vi "Personality Test.vi"(0 "GEA2 Reference In":refnum<k24>, 5 "Model":string, 11 "error in (no error)":errorcluster) -> (3 "Personality":u8, 4 "GEA2 Reference Out":refnum<k24>, 6 "Report Text":string, 8 "Pass/Fail?":bool=TRUE, 10 "Model ID":u8, 14 "Version":string, 15 "Error Out":errorcluster)   [LabVIEW 2016]
doc: "This VI performs the personality test on the control. It reads the current personality stored and compares it to the expected personality for that particular model number. If they differ then it writes to change the model number to match the expected."
uses:
  C:/Automation/DLLs/PC Dot Net/GeaCommunication.dll
  Automation/DLLs/PC Dot Net/GeaCommunication.dll
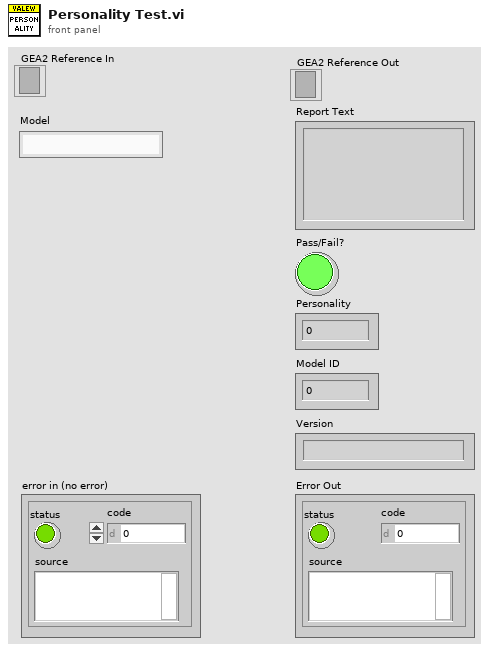
[diagram p1: front panel]
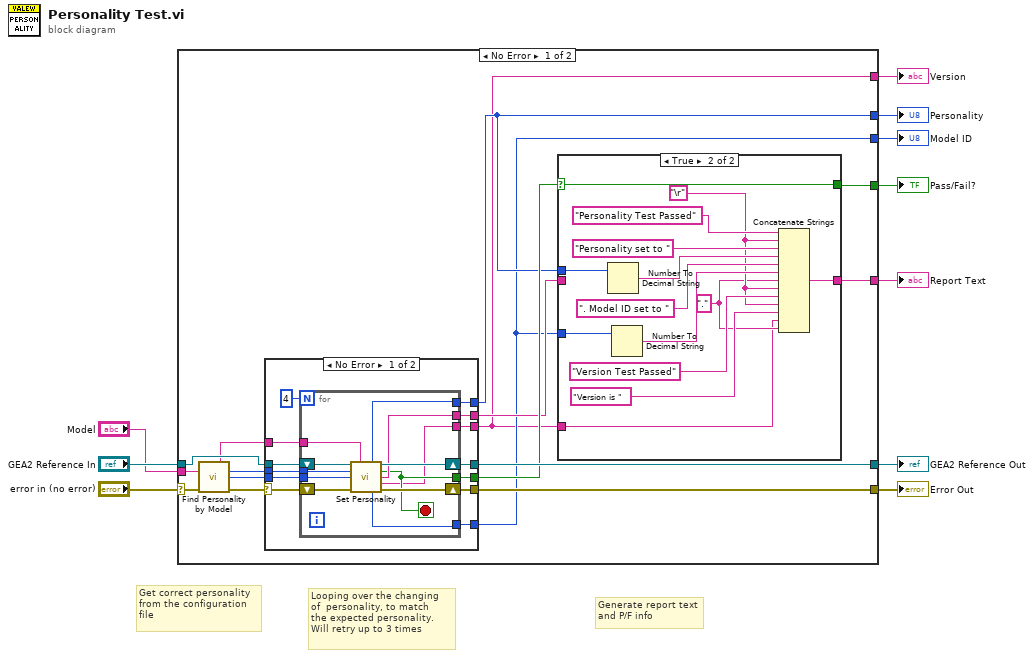
[diagram p0: block diagram]
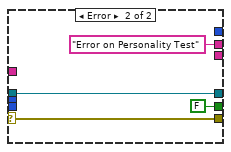
[diagram p2: hidden frame]
diagram:
  # "Generate report text\nand P/F info"
  # "Looping over the changing\nof  personality, to match \nthe expected personality. \nWill retry up to 3 times"
  # "Get correct personality\nfrom the configuration\nfile"
  n1 = case shown="No Error" "error in (no error)" {
    selector: "error in (no error)" -> [w18 w73]
    tunnel: [w26 w73] -> w10
    tunnel: "GEA2 Reference In" -> [w25 w72]
    tunnel: [w24 w72] -> w8
    tunnel: "Model" -> [w23 _]
    tunnel: [w20 _] -> w6
    tunnel: [w19 _] -> w5
    tunnel: [w13 _] -> w3
    tunnel: [w12 _] -> w1
    tunnel: [w11 _] -> w2
    frame No Error {
      n2 = call "Find Personality by Model.vi"("Model"=w23, "error in (no error)"=w18) -> ("Version"=w14:string, "Personality"=w16:u8, "Model ID"=w15:u8, "error out"=w17:errorcluster)  [unwired: 10 in]
      n3 = case shown="No Error" w17 {
        selector: w17 -> [w31 w55]
        tunnel: [w39 w55] -> w26
        tunnel: w25 -> [w38 w53]
        tunnel: [w37 w53] -> w24
        tunnel: [w35 FALSE ("Pass/Fail?")] -> w22
        tunnel: [w34 "Error on Personality Test" ("Report Text")] -> w21
        tunnel: w16 -> [w33 _]
        tunnel: w15 -> [w32 _]
        tunnel: w14 -> [w30 _]
        tunnel: [w29 _] -> w11
        tunnel: [w28 _] -> w13
        tunnel: [w27 _] -> w12
        frame No Error {
          n4 = for {
            N: 4 -> [_]
            tunnel: w33 -> [w51]
            tunnel: [w45] -> w35
            shift-right: [w49] -> w39
            shift-left: w31 -> [w50]
            shift-right: [w47] -> w37
            shift-left: w38 -> [w48]
            tunnel: [w46] -> w34
            tunnel: w32 -> [w44]
            tunnel: w30 -> [w43]
            tunnel: [w42] -> w29
            tunnel: [w41] -> w28
            tunnel: [w40] -> w27
            stop <- w45 stop-if-true
            n5 = call "Set Personality.vi"("GEA2 Reference In"=w48, "Expected Version"=w43, "Expected Personality"=w51, "Expected Model ID"=w44, "Error In"=w50) -> ("Actual Personality"=w41:u8, "GEA2 Reference Out"=w47:refnum<k24>, "Pass/Fail?"=w45:bool, "Report Text"=w46:string, "Actual Version"=w42:string, "Actual Model ID"=w40:u8, "Error Out"=w49:errorcluster)  [unwired: 4 in]
          }
        }
        frame Error {
        }
      }
      n6 = case shown="True" w22 {
        selector: w22 -> [w57 w71]
        tunnel: [w57 w71] -> w19
        tunnel: [w56 w69] -> w20
        tunnel: w21 -> [w56 _]
        tunnel: w13 -> [_ w65]
        tunnel: w12 -> [_ w64]
        tunnel: w11 -> [_ w58]
        frame False {
        }
        frame True {
          w59 = "." ("string")
          w61 = "\r"
          n7 = Number To Decimal String(number=w65) -> (decimal integer string=w67:string)  [unwired: 1 in]
          n8 = Number To Decimal String(number=w64) -> (decimal integer string=w63:string)  [unwired: 1 in]
          n9 = Concatenate Strings("Personality Test Passed", w61, "Personality set to " ("string"), w67, ". Model ID set to " ("string"), w63, w59, w61, "Version Test Passed", w61, "Version is ", w58, w59) -> (w69:string)
        }
      }
    }
    frame Error {
    }
  }
  "Error Out" <- w10
  "GEA2 Reference Out" <- w8
  "Pass/Fail?" <- w5
  "Report Text" <- w6
  "Personality" <- w3
  "Model ID" <- w1
  "Version" <- w2
